vi "Update_3D_Mesh.vi"(7 "3D Plot Data":T1, 8 "Z (GRID)":dbl[][](array[numeric])=[[0.0, 0.0, 0.0, 309.7599999999984, 309.7599999999984, 0.0, 0.0, 0.0], [0.0, 309.76000000000204, 619.5200000000004, 309.7600000000002, 619.5200000000004, 309.7600000000002, 0.0, 309.76000000000204], [0.0, 619.5200000000004, 2787.84, 1548.7999999999993, 929.2799999999988, 929.2800000000025, 309.76000000000204, 309.7599999999984], [0.0, 309.7599999999984, 1239.0400000000009, 2478.0800000000017, 3097.600000000002, 1548.7999999999993, 929.2799999999988, 619.5200000000004], [0.0, 0.0, 619.5200000000004, 929.2799999999988, 1239.0400000000009, 1239.0399999999972, 929.2799999999988, 309.76000000000204], [0.0, 0.0, 309.76000000000204, 309.7599999999984, 619.5200000000004, 619.5200000000004, 309.76000000000204, 309.76000000000204], [0.0, 0.0, 0.0, 0.0, 0.0, 0.0, 309.76000000000204, 309.7599999999984], [0.0, 0.0, 0.0, 0.0, 0.0, 0.0, 309.7599999999984, 0.0]], 9 "Y (GRID)":dbl[][](array[numeric])=[[3.7549999999996544, 6.008000000000038, 12.766999999999996, 30.791000000000167, 18.023999999999887, 0.0, -15.770999999999958, -13.518000000000029], [10.51400000000001, -9.763000000000034, 47.31299999999993, 85.6139999999998, 93.1239999999998, 52.570000000000164, 12.766999999999825, -12.015999999999622], [22.529999999999973, 60.07999999999993, 46.56200000000001, 295.894, -3.7550000000000026, -18.77500000000009, 36.79899999999998, -67.58999999999997], [6.008000000000038, 23.28099999999995, 44.309, -155.457, 31.542, -218.541, 25.534000000000106, 5.257000000000062], [2.252999999999986, -3.0039999999999054, -74.34900000000016, 3.7549999999999955, -9.76299999999992, -72.84700000000001, 17.27299999999991, -82.61], [19.52600000000075, -1.5019999999999527, -72.84700000000066, -46.5619999999999, -83.36099999999988, -90.11999999999989, -46.56200000000001, -46.5619999999999], [11.265, -4.5060000000000855, -40.55400000000009, -6.0079999999999245, 7.510000000000019, 6.0079999999999245, 9.011999999999944, -18.024], [-0.7509999999992942, 13.518000000000029, -2.253, 6.00800000000072, 0.7510000000002037, -11.265000000000327, -18.77500000000009, -8.260999999999967]], 10 "X (GRID)":dbl[][](array[numeric])=[[36.048, 13.518000000000029, 26.285000000000082, 40.55400000000009, 22.529999999999745, 39.803, 24.783000000000015, 12.766999999999825], [27.035999999999998, 57.07600000000002, -16.522000000000048, 171.97900000000027, 122.41300000000001, 135.93099999999959, 114.90300000000025, 21.778999999999996], [14.269000000000005, 3.7549999999999955, 817.0879999999997, 467.1219999999994, 445.34299999999985, 379.2550000000001, 228.3040000000001, 99.1319999999996], [-2.2529999999997017, -50.31700000000001, -25.533999999999992, -117.15599999999995, -596.2940000000003, 227.55299999999988, -26.284999999999854, 83.36099999999988], [-9.012, 25.534000000000106, -40.55400000000009, 115.654, -18.023999999999887, 5.257000000000062, 208.77799999999934, 147.1959999999999], [-23.28099999999995, -17.27299999999991, 13.518000000000029, 10.51400000000001, 28.53800000000001, 22.529999999999973, 57.82699999999977, 97.63000000000011], [-18.023999999999887, -29.289000000000215, -12.015999999999622, 0.0, 15.019999999999527, 34.54599999999982, 45.05999999999949, 29.28899999999976], [-21.027999999999793, -24.031999999999698, -24.7829999999999, 13.518000000000029, 11.264999999999986, 18.023999999999432, 6.008000000000266, -0.7510000000002037]], 11 "SceneDrawable in":refnum<vi>) -> (3 "SceneDrawable out":refnum<vi>)   [LabVIEW 2016]
uses:
  controls/3D_Plot_Data.ctl
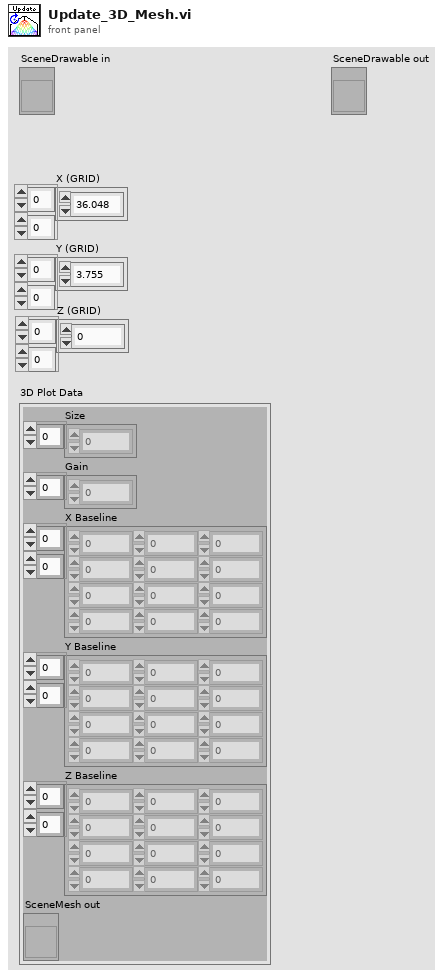
[diagram p1: front panel]
types:
  T1 = typedef "3D_Plot_Data.ctl" = cluster{"Size":i32[], "Gain":dbl[], "X Baseline":dbl[][], "Y Baseline":dbl[][], "Z Baseline":dbl[][], "SceneMesh out":refnum<vi>}
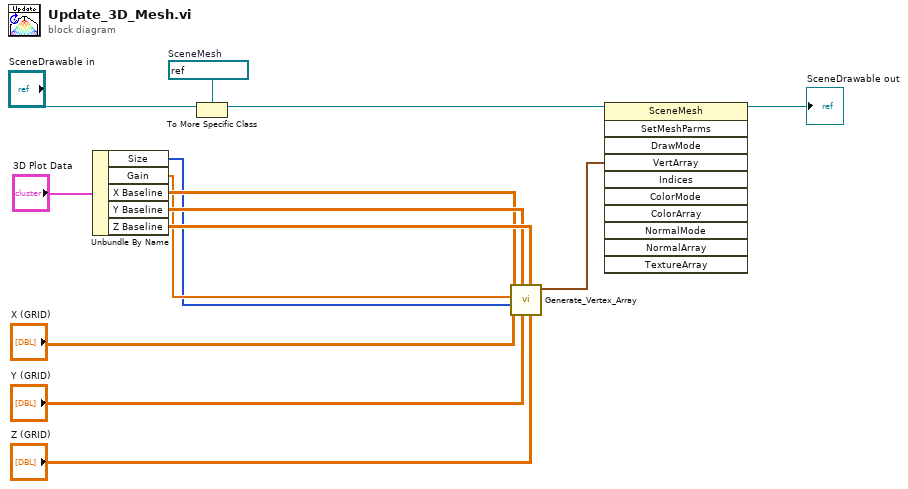
[diagram p0: block diagram]
diagram:
  w11 = refnum<vi> refnum  # SceneMesh
  n1 = Unbundle By Name("3D Plot Data") -> ("Size"=w1:i32[], "Gain"=w2:dbl[], "X Baseline"=w3:dbl[][], "Y Baseline"=w4:dbl[][], "Z Baseline"=w5:dbl[][])
  n2 = To More Specific Class(target class=w11, reference="SceneDrawable in") -> (specific class reference=w13:refnum<vi>)  [unwired: 1 in, 1 out]
  n3 = call "Generate_Vertex_Array.vi"("Sensor Z"="Z (GRID)", "Z Baseline"=w5, "Sensor Y"="Y (GRID)", "Y Baseline"=w4, "Sensor X"="X (GRID)", "Size"=w1, "Gain"=w2, "X Baseline"=w3) -> ("Init Vertex Array"=w7:cluster{"x":dbl, "y":dbl, "z":dbl}[])  [unwired: 3 in]
  n4 = invoke class="SceneMesh" method="SetMeshParms"(reference=w13, "VertArray"=w7) -> (reference out=→"SceneDrawable out":refnum<vi>)  [unwired: 9 in, 10 out]
